vi "8. FGV Cksum check.vi"(8 "error in (no error)":errorcluster, 10 "Calculated cksum":u32=500, 11 "VISA resource name":refnum<visa-resource-name>="COM3") -> (0 "error out":errorcluster, 3 "Cksum":u32)   [LabVIEW 2014]
uses:
  control/FGV Serial Tasks.ctl
panel:
  out "Different?":bool
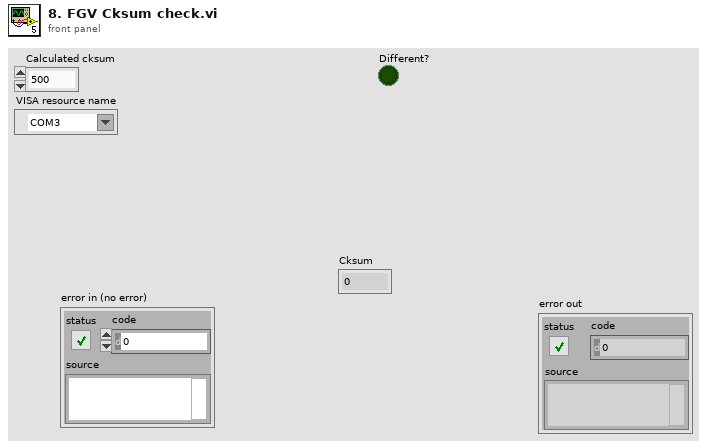
[diagram p1: front panel]
types:
  T1 = typedef "FGV Serial Tasks.ctl" = enum16{"Open", "Read", "Write", "Close", "Flush"}
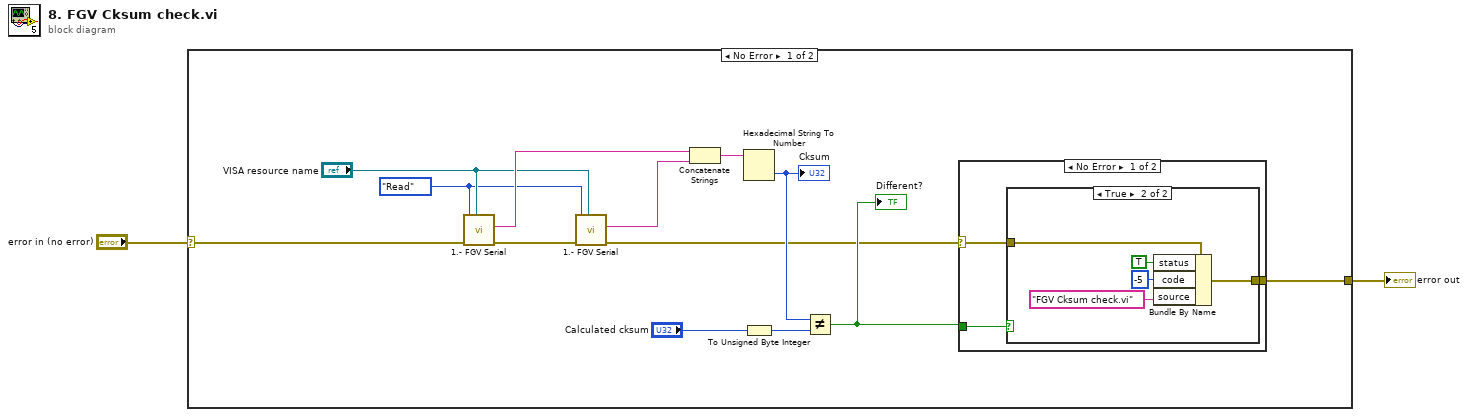
[diagram p0: block diagram]
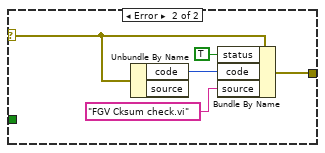
[diagram p3: hidden frame]
diagram:
  n1 = case shown="No Error" "error in (no error)" {
    selector: "error in (no error)" -> [w13 w30]
    tunnel: [w6 w30] -> w1
    frame No Error {
      w3 = FGV_Serial_Tasks."Read" ("Task")
      n2 = call "1.- FGV Serial.vi"("VISA resource name"="VISA resource name", "error in (no error)"=w13, "Task"=w3) -> ("error out"=w14:errorcluster, "Receive buffer"=w15:string)  [unwired: 6 in, 1 out]
      n3 = call "1.- FGV Serial.vi"("VISA resource name"="VISA resource name", "error in (no error)"=w14, "Task"=w3) -> ("error out"=w7:errorcluster, "Receive buffer"=w4:string)  [unwired: 6 in, 1 out]
      n4 = Concatenate Strings(w15, w4) -> (w12:string)
      n5 = Hexadecimal String To Number(string=w12) -> (number=w11:u32)  [unwired: 2 in, 1 out]
      "Cksum" <- w11
      n6 = To Unsigned Byte Integer(number="Calculated cksum") -> (unsigned 8bit integer=w9:u8)
      n7 = Not Equal?(x=w11, y=w9) -> (x != y?=w8:bool)
      "Different?" <- w8
      n8 = case shown="No Error" w7 {
        selector: w7 -> [w16 w25]
        tunnel: w8 -> [w18 _]
        tunnel: [w17 w26] -> w6
        frame No Error {
          n9 = case shown="True" w18 {
            tunnel: [w19 w24] -> w17
            tunnel: w16 -> [w19 w23]
            frame False {
            }
            frame True {
              n10 = Bundle By Name(cluster=w23, "status"=TRUE, "code"=-5, "source"="FGV Cksum check.vi") -> (w24:errorcluster)
            }
          }
        }
        frame Error {
          n11 = Unbundle By Name(w25) -> ("code"=w29:i32)  [unwired: 1 out]
          n12 = Bundle By Name(cluster=w25, "status"=TRUE, "code"=w29, "source"="FGV Cksum check.vi") -> (w26:errorcluster)
        }
      }
    }
    frame Error {
    }
  }
  "error out" <- w1
